vi "Actor Core.vi"(8 "error in":errorcluster, 11 "Import Export in":refnum<class "Export.lvclass">) -> (0 "error out":errorcluster, 3 "Actor out":refnum<class "Actor.lvclass">)   [LabVIEW 2023, in "Data Analysis.lvlib" / "Export.lvlib" / "Export.lvclass"]
doc: "(<B>Filename</B>: Actor Framework.lvlib:Actor.lvclass:Actor Core.vi)\n\nReceives messages to the actor, reacts to them, and initiates any error handling that may shut the actor down.\n\nDescendant classes may override this VI to append parallel tasks for the actor to complete while it handles messages. Overrides use the Call Parent Class Method node."
uses:
  Export.lvclass
  C:/Program Files/National Instruments/LabVIEW 2023/vi.lib/ActorFramework/Actor/Actor.lvclass
  <vilib>/ActorFramework/Actor/Actor.lvclass
  Export.lvclass/Export.ctl
  <vilib>/ActorFramework/Actor/Actor.lvclass/Actor.ctl
  <vilib>/ActorFramework/Message Enqueuer/Message Enqueuer.lvclass/Message Enqueuer.ctl
  Subpanel-Abstract Messages/Insert SP Msg/Insert SP Msg.lvclass/Insert SP Msg.ctl
  Import Export Messages/Show Tables Msg/Show Tables Msg.lvclass/Show Tables Msg.ctl
  Import Export Messages/Show the data Msg/Show the data Msg.lvclass/Show the data Msg.ctl
  Import Export Messages/Export the Data Msg/Export the Data Msg.lvclass/Export the Data Msg.ctl
  <vilib>/ActorFramework/Message Enqueuer/Init from Existing Queue.vi
  <vilib>/ActorFramework/Message Enqueuer/Enqueue.vi
  Subpanel-Abstract Messages/Insert SP Msg/Insert SP Msg.lvclass
  C:/Program Files/National Instruments/LabVIEW 2023/vi.lib/ActorFramework/Message/Message.lvclass
  Import Export Messages/Show Tables Msg/Show Tables Msg.lvclass
  Import Export Messages/Show the data Msg/Show the data Msg.lvclass
  Import Export Messages/Export the Data Msg/Export the Data Msg.lvclass
  <vilib>/ActorFramework/Message Priority Queue/Priority Enqueue.vi
  <vilib>/ActorFramework/Message Enqueuer/Message Enqueuer.lvclass
  Subpanel-Abstract/Subpanel-Abstract.lvclass
panel:
  in  "File Format":string(combo)="XLS"
  in  "Table Names":string(combo)
  in  "Export":bool
  in  "Data":i32(listbox)=-1
  in  "Stop":bool
  # "One Combo Box- Show all the Tables for Selected Schema.\n2. Export Option Enable FE, FF Actor to"
  # "Export Data"
  # "*Non of above  filters are applicable here"
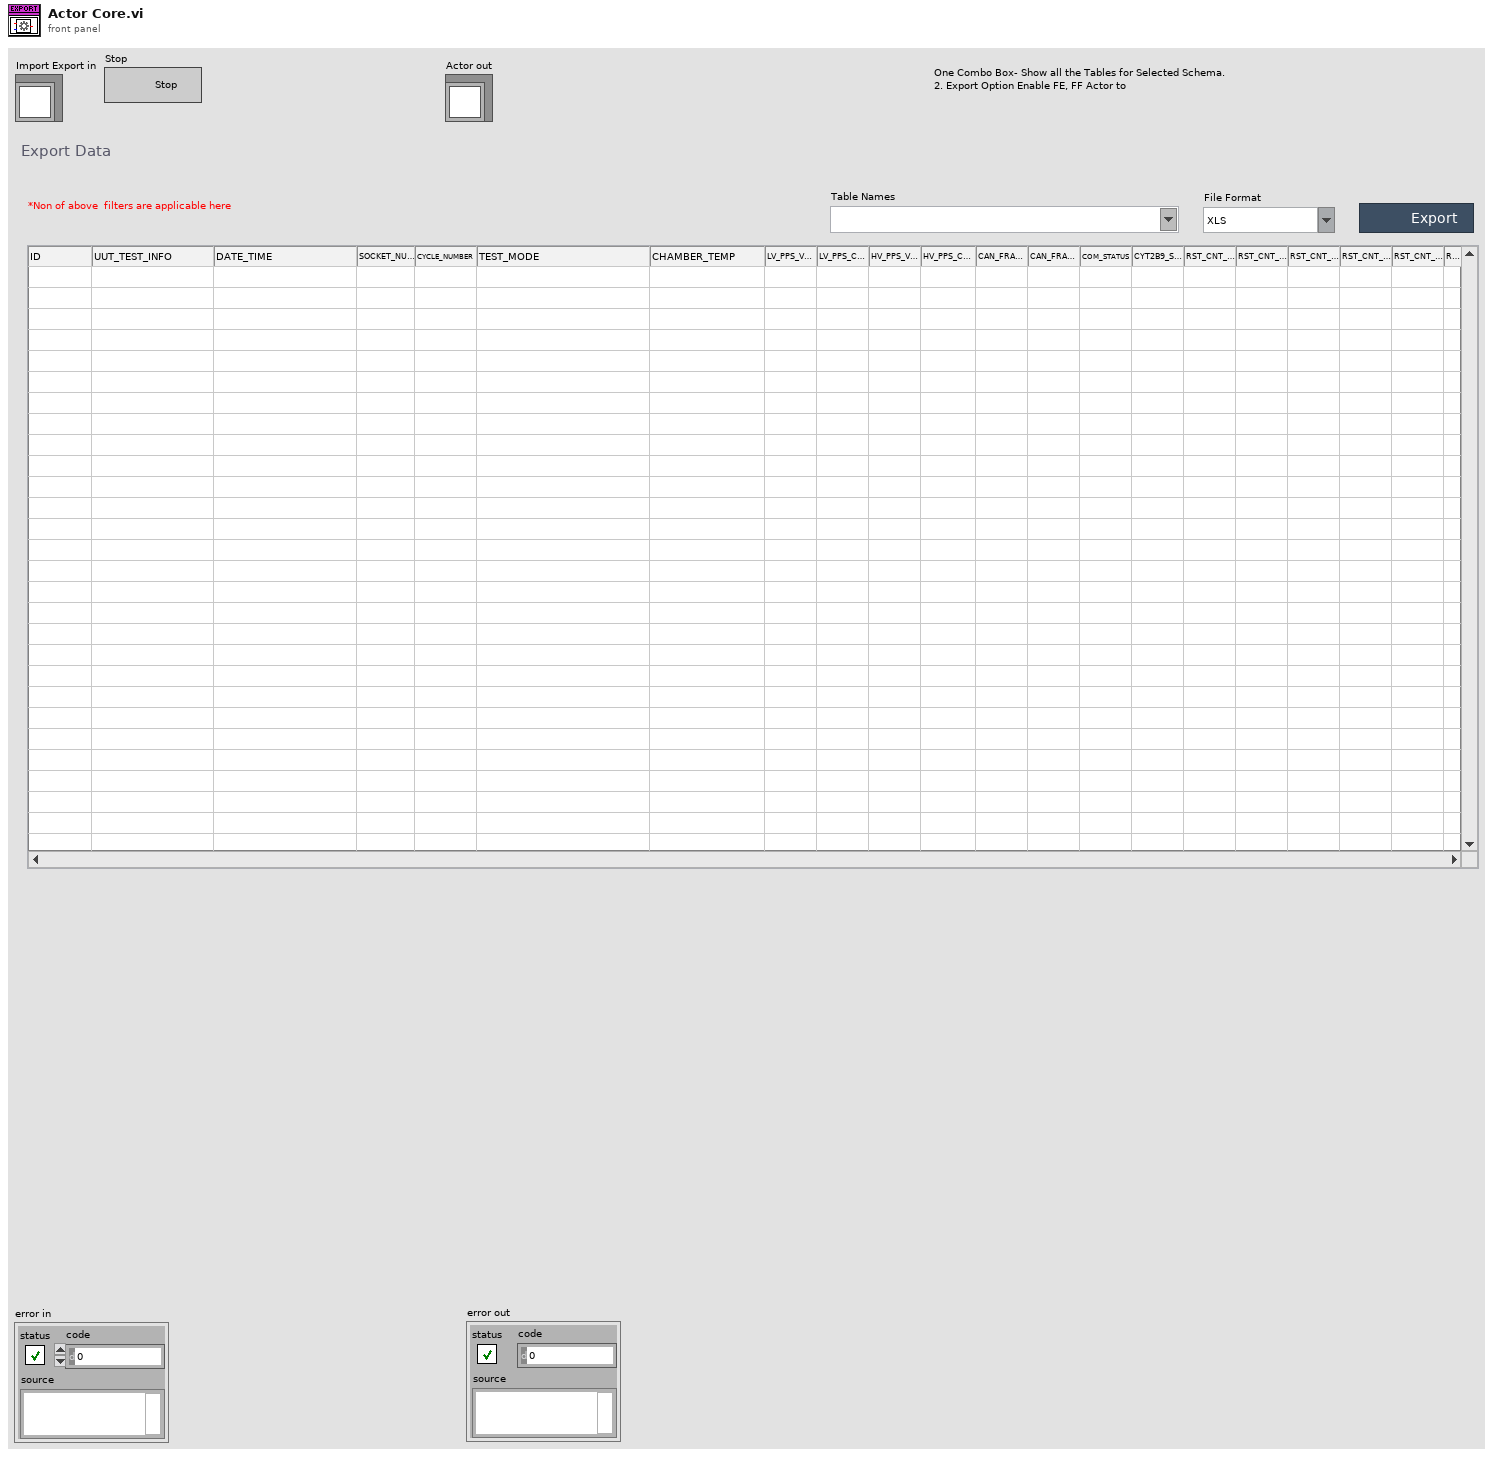
[diagram p1: front panel]
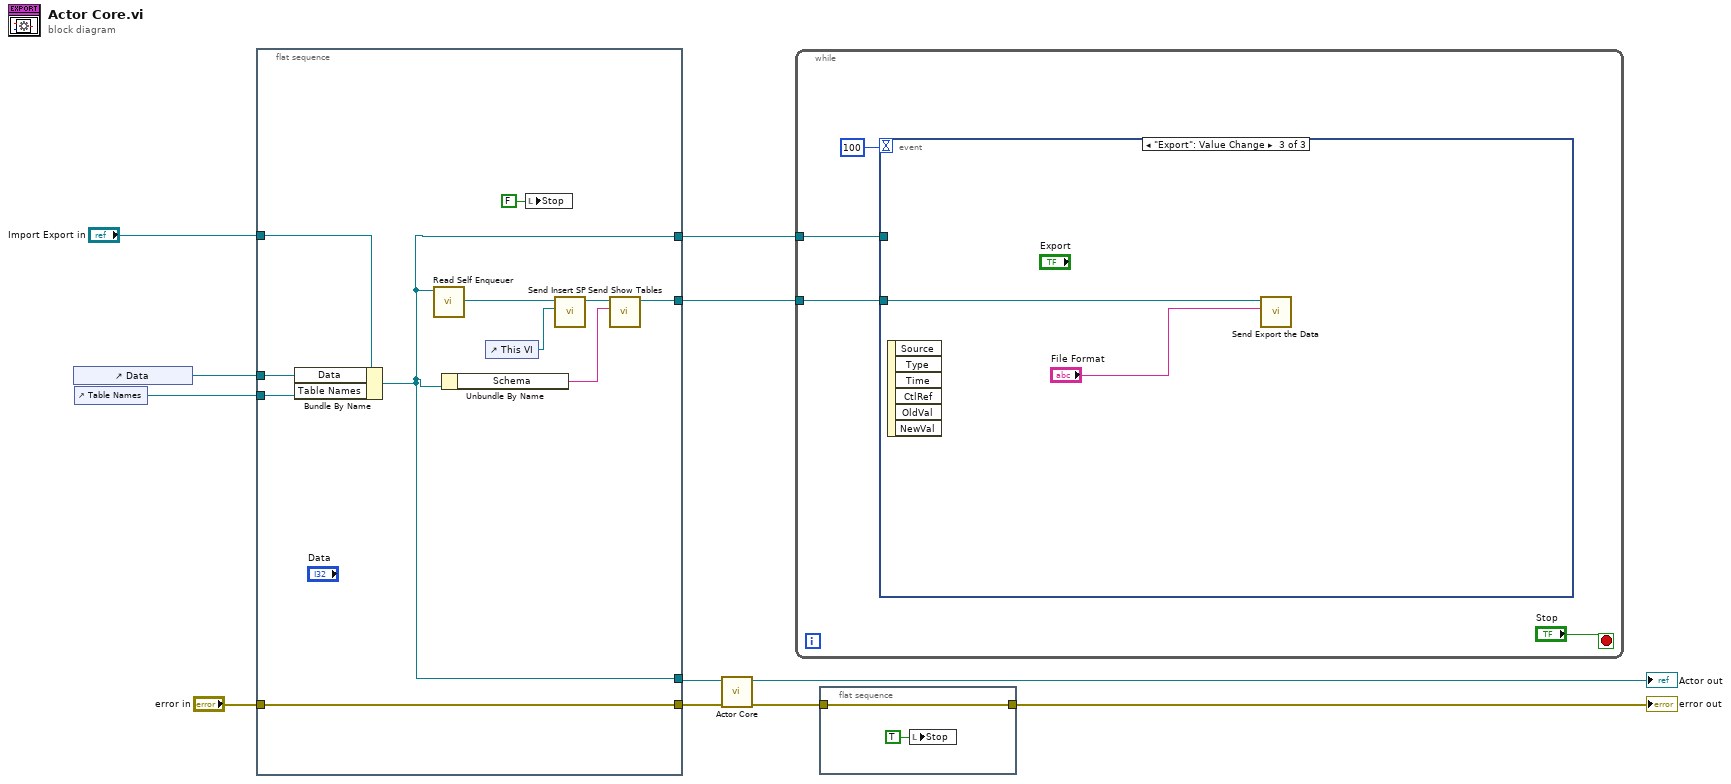
[diagram p0: block diagram]
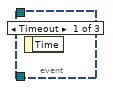
[diagram p2: hidden frame]
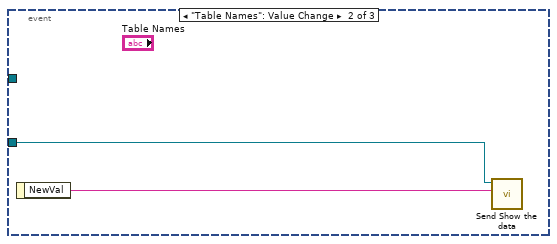
[diagram p3: hidden frame]
diagram:
  n1 = control-ref of="Data"() -> (w2:refnum<vi>)
  n2 = control-ref of="Table Names"() -> (w1:refnum<vi>)
  n3 = flat-sequence {
    tunnel: "error in" -> [w22]
    tunnel: [w22] -> w9
    tunnel: "Import Export in" -> [w18]
    tunnel: [w13] -> w7
    tunnel: [w14] -> w6
    tunnel: [w13] -> w5
    tunnel: w2 -> [w17]
    tunnel: w1 -> [w16]
    frame #0 {
      n4 = Bundle By Name(cluster=w18, "Data"=w17, "Table Names"=w16) -> (w13:refnum<class "Export.lvclass">)
      n5 = call <vilib>:"Read Self Enqueuer.vi"("Actor"=w13) -> ("Self Enqueuer"=w20:refnum<class "Message Enqueuer.lvclass">)  [unwired: 10 in]
      n6 = Unbundle By Name(w13) -> ("Schema"=w12:string)
      n7 = control-ref of="This VI"() -> (w19:refnum<vi>)
      n8 = local write "Stop"(FALSE ("Stop")) -> ()
      n9 = call "Send Insert SP.vi"("VI Ref"=w19, "Message Enqueuer"=w20) -> ("Message Enqueuer out"=w15:refnum<class "Message Enqueuer.lvclass">)  [unwired: 8 in, 1 out]
      n10 = call "Send Show Tables.vi"("Report Data.Schema"=w12, "Message Enqueuer"=w15) -> ("Message Enqueuer out"=w14:refnum<class "Message Enqueuer.lvclass">)  [unwired: 8 in, 1 out]
    }
  }
  n11 = call-parent "Actor Core.vi"("error in"=w9, "Actor in"=w7) -> ("error out"=w4:errorcluster, "Actor out"=→"Actor out":refnum<class "Actor.lvclass">)  [unwired: 8 in]
  n12 = while {
    tunnel: w6 -> [w24]
    tunnel: w5 -> [w23]
    stop <- "Stop" stop-if-true
    n13 = event shown="[2] \"Export\": Value Change" {
      selector: _ -> [_ _ _]
      dyn-events: _ -> [_ _ _]
      timeout: 100 -> [_ _ _]
      tunnel: w24 -> [_ w28 w30]
      tunnel: w23 -> [_ _ _]
      event Timeout {
        n14 = event-data() -> ()  [unwired: 1 in, 1 out]
      }
      event "Table Names": Value Change {
        n15 = event-data() -> ("NewVal"=w27:string)  [unwired: 1 in]
        n16 = call "Send Show the data.vi"("Table Name"=w27, "Message Enqueuer"=w28) -> ()  [unwired: 8 in, 2 out]
      }
      event "Export": Value Change {
        n17 = event-data() -> ()  [unwired: 1 in, 6 out]
        n18 = call "Send Export the Data.vi"("File Format"="File Format", "Message Enqueuer"=w30) -> ()  [unwired: 8 in, 2 out]
      }
    }
  }
  n19 = flat-sequence {
    tunnel: w4 -> [w32]
    tunnel: [w32] -> w3
    frame #0 {
      n20 = local write "Stop"(TRUE ("Stop")) -> ()
    }
  }
  "error out" <- w3
